vi "Main.vi"   [LabVIEW 2013]
types:
  T1 = enum16{"open", "replace", "create", "open or create", "replace or create", "replace or create with confirmation"}
  T2 = cluster{"Team Number":string, "Autonomous Comments":string, "Autonomous?":string, "Did they pick up more discs?":string, "1 Point":dbl, "2 Points":dbl, "3 Points":dbl}
  T3 = cluster{"1 Point":dbl, "2 Points":dbl, "3 Points":dbl, "5 Points":dbl, "Where do they pick up discs?":string, "Comments":string, "Missed Shots":dbl, "Pyramid":string, "Total":dbl}
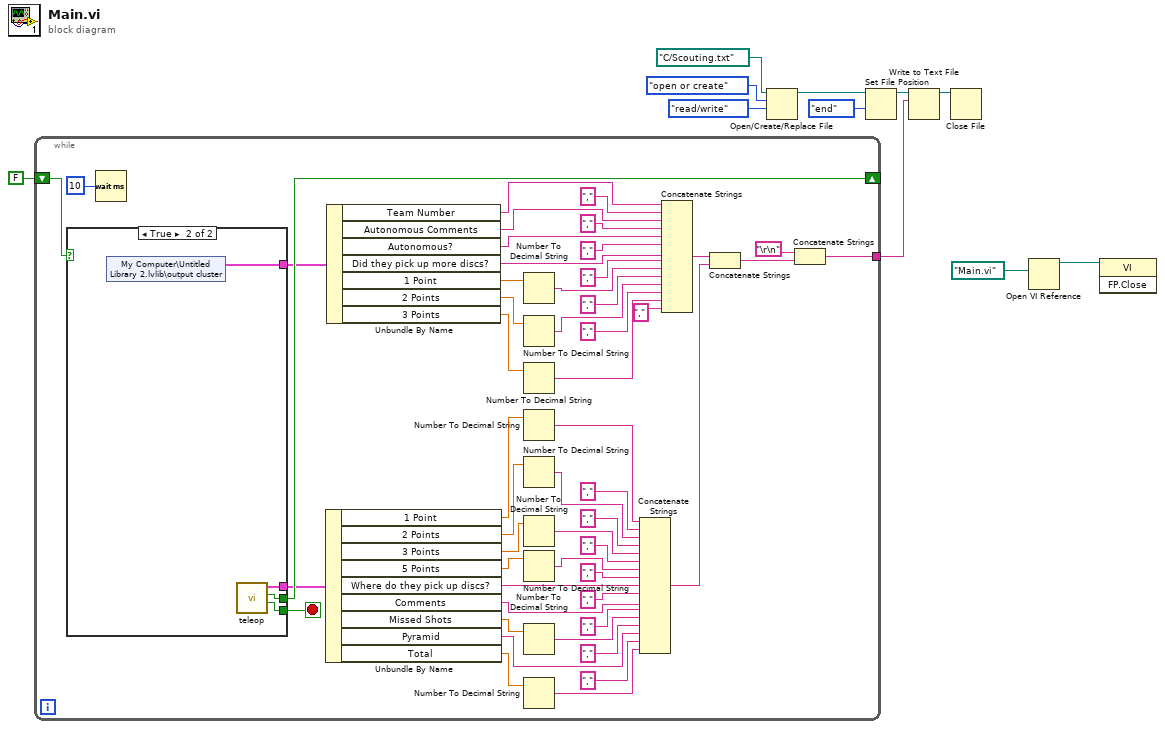
[diagram p0: block diagram]
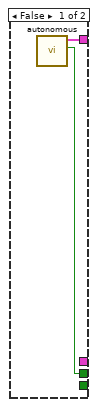
[diagram p2: hidden frame]
diagram:
  n1 = while {
    shift-right: [w61] -> _
    shift-left: FALSE ("Boolean") -> [w62]
    tunnel: [w48] -> w3
    stop <- w59 stop-if-true
    n2 = case shown="True" w62 {
      tunnel: [w64 w68] -> w61
      tunnel: [_ w67] -> w59
      tunnel: [w63 w66] -> w31
      tunnel: [_ w65] -> w21
      frame False {
        n3 = call "autonomous.vi"() -> ("Switch to teleop"=w64:bool, "output cluster"=w63:T2)  [unwired: 8 in]
      }
      frame True {
        n4 = shared-variable "My Computer\\Untitled Library 2.lvlib\\output cluster"() -> (w66:T2)  [unwired: 1 in, 1 out]
        n5 = call "teleop.vi"() -> ("Stop program and write to file"=w67:bool, "SWITCH TO AUTONOMOUS"=w68:bool, "output cluster"=w65:T3)  [unwired: 7 in]
      }
    }
    n6 = Wait (ms)(milliseconds to wait=u32 10) -> ()  [unwired: 1 out]
    n7 = Unbundle By Name(w21) -> ("1 Point"=w20:dbl, "2 Points"=w19:dbl, "3 Points"=w18:dbl, "5 Points"=w17:dbl, "Where do they pick up discs?"=w16:string, "Comments"=w15:string, "Missed Shots"=w14:dbl, "Pyramid"=w13:string, "Total"=w12:dbl)
    n8 = Unbundle By Name(w31) -> ("Team Number"=w30:string, "Autonomous Comments"=w29:string, "Autonomous?"=w25:string, "Did they pick up more discs?"=w24:string, "1 Point"=w28:dbl, "2 Points"=w27:dbl, "3 Points"=w26:dbl)
    n9 = Number To Decimal String(number=w28) -> (decimal integer string=w49:string)  [unwired: 1 in]
    n10 = Number To Decimal String(number=w27) -> (decimal integer string=w50:string)  [unwired: 1 in]
    n11 = Number To Decimal String(number=w26) -> (decimal integer string=w51:string)  [unwired: 1 in]
    n12 = Number To Decimal String(number=w20) -> (decimal integer string=w47:string)  [unwired: 1 in]
    n13 = Number To Decimal String(number=w19) -> (decimal integer string=w46:string)  [unwired: 1 in]
    n14 = Number To Decimal String(number=w18) -> (decimal integer string=w45:string)  [unwired: 1 in]
    n15 = Number To Decimal String(number=w17) -> (decimal integer string=w44:string)  [unwired: 1 in]
    n16 = Number To Decimal String(number=w14) -> (decimal integer string=w43:string)  [unwired: 1 in]
    n17 = Number To Decimal String(number=w12) -> (decimal integer string=w22:string)  [unwired: 1 in]
    n18 = Concatenate Strings(w47, "," ("string"), w46, "," ("string"), w45, "," ("string"), w44, "," ("string"), w16, "," ("string"), w15, "," ("string"), w43, "," ("string"), w13, "," ("string"), w22) -> (w34:string)
    n19 = Concatenate Strings(w30, "," ("string"), w29, "," ("string"), w25, "," ("string"), w24, "," ("string"), w49, "," ("string"), w50, "," ("string"), w51, "," ("string")) -> (w35:string)
    n20 = Concatenate Strings(w35, w34) -> (w33:string)
    n21 = Concatenate Strings("\r\n", w33) -> (w48:string)
  }
  n22 = Open/Create/Replace File(file path (use dialog)=path "C:/Scouting.txt", operation (0:open)=T1."open or create", access (0:read/write)=enum16{"read/write", "read-only", "write-only"}."read/write") -> (refnum out=w5:refnum<file>)  [unwired: 3 in, 2 out]
  n23 = Set File Position(refnum=w5, from (0:start)=enum16{"start", "end", "current"}."end") -> (refnum out=w4:refnum<file>)  [unwired: 2 in, 1 out]
  n24 = Write to Text File(file (use dialog)=w4, text=w3) -> (refnum out=w7:refnum<file>)  [unwired: 2 in, 2 out]
  n25 = Close File(refnum=w7) -> ()  [unwired: 1 in, 2 out]
  n26 = Open VI Reference(vi path=path "Main.vi") -> (vi reference=w1:refnum<vi>)  [unwired: 5 in, 1 out]
  n27 = invoke class="VI" method="FP.Close"(reference=w1) -> ()  [unwired: 2 in, 3 out]
